vi "_Get Experiment List.vi"(4 "error in (no error)":errorcluster, 7 "node in":refnum<k20>) -> (0 "error out":errorcluster, 1 "ExptParamAndMR":T2(array[cluster]), 2 "Expt":string[][](array[string]), 3 "node out":refnum<k20>)   [LabVIEW 2015]
uses:
  Type/_Mass Range Parameters.ctl
  Server/AutoCal/Controls/xml Parameter Type.ctl
  <vilib>/xml/Close Reference(Node).vi
  <vilib>/xml/NI_XML.lvlib
panel:
  # "Num             Type            Polarity        StartTime      StopTime        Cycles       PauseTime    DelayTime          MR#         DwellTime   Comment"
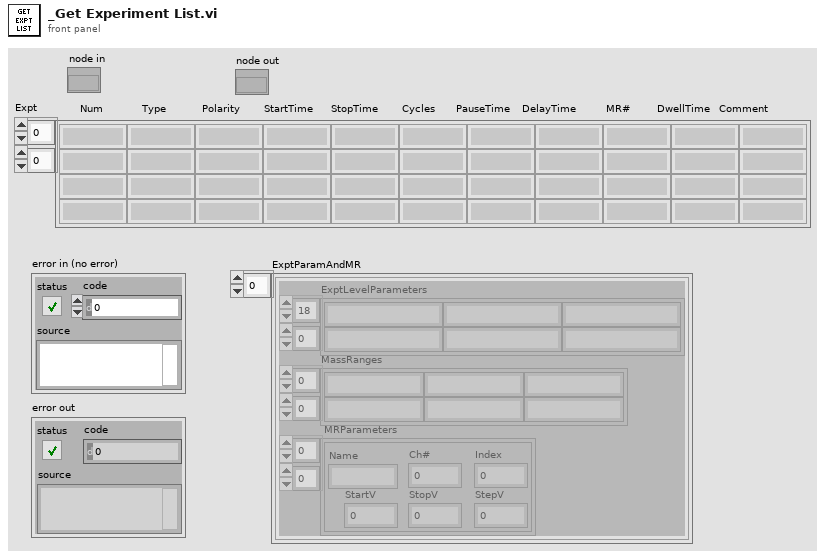
[diagram p1: front panel]
types:
  T1 = typedef "_Mass Range Parameters.ctl" = cluster{"Name":string, "Ch#":u8, "StartV":dbl, "StopV":dbl, "StepV":dbl, "Index":u8}
  T2 = cluster{"ExptLevelParameters":string[][], "MassRanges":string[][], " MRParameters":T1[][]}[]
  T3 = typedef "xml Parameter Type.ctl" = enum16{"Method Parameters", "Experiment Parameters"}
  T4 = cluster{"Parameters List":string[][], "Mass Ranges":string[][], " MRParameters":T1[][]}
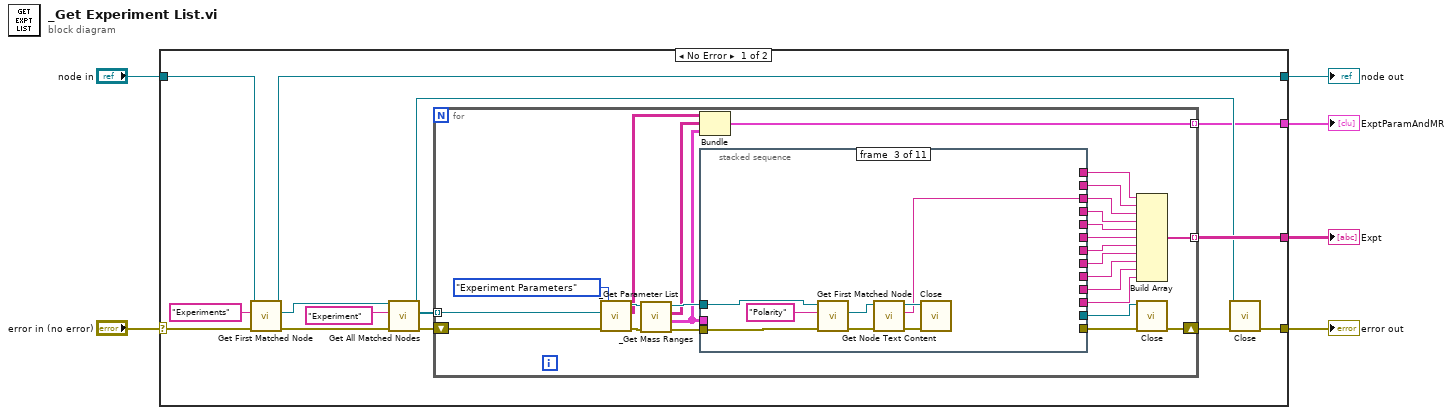
[diagram p0: block diagram]
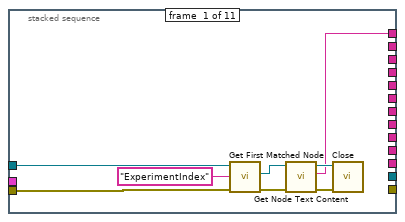
[diagram p2: hidden frame]
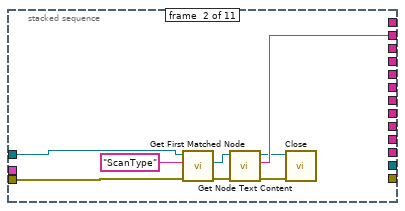
[diagram p3: hidden frame]
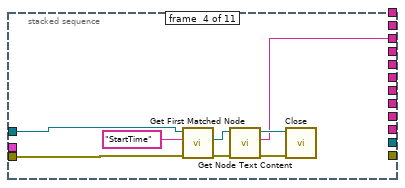
[diagram p4: hidden frame]
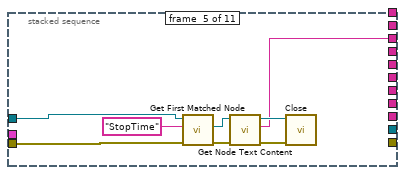
[diagram p5: hidden frame]
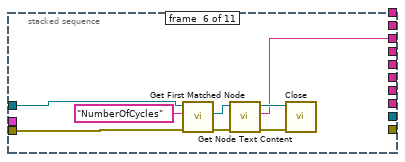
[diagram p6: hidden frame]
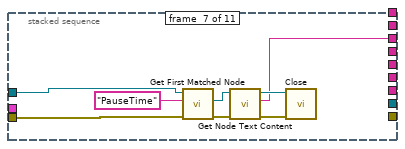
[diagram p7: hidden frame]
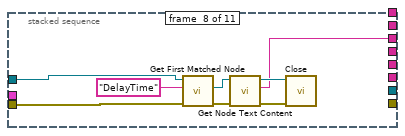
[diagram p8: hidden frame]
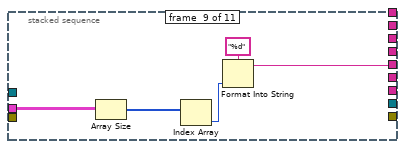
[diagram p9: hidden frame]
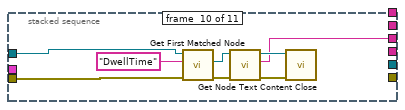
[diagram p10: hidden frame]
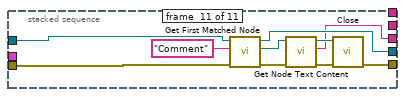
[diagram p11: hidden frame]
diagram:
  n1 = case shown="No Error" "error in (no error)" {
    selector: "error in (no error)" -> [w18 w135]
    tunnel: [w19 _] -> w6
    tunnel: [w9 w135] -> w5
    tunnel: "node in" -> [w16 w134]
    tunnel: [w15 w134] -> w2
    tunnel: [w7 _] -> w1
    frame No Error {
      n2 = call <vilib>:"Get First Matched Node.vi"("error in (no error)"=w18, "XPath expression"="Experiments", "node in"=w16) -> ("error out"=w17:errorcluster, "node result"=w13:refnum<k20>, "node out"=w15:refnum<k20>)  [unwired: 6 in]
      n3 = call <vilib>:"Get All Matched Nodes.vi"("error in (no error)"=w17, "XPath expression"="Experiment", "node in"=w13) -> ("error out"=w11:errorcluster, "node result array"=w12:refnum<k20>[], "node out"=w8:refnum<k20>)  [unwired: 6 in]
      n4 = for {
        shift-right: [w46] -> w10
        shift-left: w11 -> [w30]
        tunnel: w12 -> [w31] mode=indexing
        tunnel: [w36] -> w19 mode=indexing
        tunnel: [w23] -> w7 mode=indexing
        n5 = call "_Get Parameter List.vi"("error in (no error)"=w30, "Parameter Type"=xml_Parameter_Type."Experiment Parameters", "node in"=w31) -> ("error out"=w27:errorcluster, "Parameters List"=w25:string[][], "node out"=w29:refnum<k20>)  [unwired: 2 in]
        n6 = call "_Get Mass Ranges.vi"("error in (no error)"=w27, "node in"=w29) -> ("error out"=w26:errorcluster, "MRParameters"=w21:T1[][], "Mass Ranges"=w24:string[][], "node out"=w28:refnum<k20>)  [unwired: 2 in]
        n7 = Bundle("Parameters List"=w25, "Mass Ranges"=w24, "MRParameters"=w21) -> (w23:T4)  [unwired: 1 in]
        n8 = stacked-sequence {
          tunnel: w28 -> [w54 w62 w70 w78 w86 w94 w102 w110 _ w123 w133]
          tunnel: w26 -> [w53 w61 w69 w77 w85 w93 w101 w109 _ w122 w132]
          tunnel: [w47 _ _ _ _ _ _ _ _ _ _] -> w45
          tunnel: [_ w58 _ _ _ _ _ _ _ _ _] -> w44
          tunnel: [_ _ w63 _ _ _ _ _ _ _ _] -> w43
          tunnel: [_ _ _ w71 _ _ _ _ _ _ _] -> w42
          tunnel: [_ _ _ _ w79 _ _ _ _ _ _] -> w41
          tunnel: [_ _ _ _ _ w87 _ _ _ _ _] -> w40
          tunnel: [_ _ _ _ _ _ w95 _ _ _ _] -> w39
          tunnel: [_ _ _ _ _ _ _ w103 _ _ _] -> w38
          tunnel: [_ _ _ _ _ _ _ _ w111 _ _] -> w37
          tunnel: [_ _ _ _ _ _ _ _ _ _ w130] -> w35
          tunnel: [_ _ _ _ _ _ _ _ _ _ w129] -> w34
          tunnel: [_ _ _ _ _ _ _ _ _ _ w124] -> w33
          tunnel: [_ _ _ _ _ _ _ _ _ w116 _] -> w32
          tunnel: w21 -> [_ _ _ _ _ _ _ _ w115 _ _]
          frame #0 {
            n9 = call <vilib>:"Get First Matched Node.vi"("error in (no error)"=w53, "XPath expression"="ExperimentIndex", "node in"=w54) -> ("error out"=w50:errorcluster, "node result"=w51:refnum<k20>)  [unwired: 6 in, 1 out]
            n10 = call <vilib>:"Get Node Text Content.vi"("error in (no error)"=w50, "node in"=w51) -> ("error out"=w48:errorcluster, "node text"=w47:string, "node out"=w49:refnum<k20>)  [unwired: 7 in]
            n11 = call-poly <vilib>:"Close.vi"("error in (no error)"=w48, "node"=w49) -> ()  [unwired: 7 in, 1 out]
          }
          frame #1 {
            n12 = call <vilib>:"Get First Matched Node.vi"("error in (no error)"=w61, "XPath expression"="ScanType", "node in"=w62) -> ("error out"=w55:errorcluster, "node result"=w59:refnum<k20>)  [unwired: 6 in, 1 out]
            n13 = call <vilib>:"Get Node Text Content.vi"("error in (no error)"=w55, "node in"=w59) -> ("error out"=w56:errorcluster, "node text"=w58:string, "node out"=w57:refnum<k20>)  [unwired: 7 in]
            n14 = call-poly <vilib>:"Close.vi"("error in (no error)"=w56, "node"=w57) -> ()  [unwired: 7 in, 1 out]
          }
          frame #2 {
            n15 = call <vilib>:"Get First Matched Node.vi"("error in (no error)"=w69, "XPath expression"="Polarity", "node in"=w70) -> ("error out"=w66:errorcluster, "node result"=w67:refnum<k20>)  [unwired: 6 in, 1 out]
            n16 = call <vilib>:"Get Node Text Content.vi"("error in (no error)"=w66, "node in"=w67) -> ("error out"=w65:errorcluster, "node text"=w63:string, "node out"=w64:refnum<k20>)  [unwired: 7 in]
            n17 = call-poly <vilib>:"Close.vi"("error in (no error)"=w65, "node"=w64) -> ()  [unwired: 7 in, 1 out]
          }
          frame #3 {
            n18 = call <vilib>:"Get First Matched Node.vi"("error in (no error)"=w77, "XPath expression"="StartTime", "node in"=w78) -> ("error out"=w74:errorcluster, "node result"=w75:refnum<k20>)  [unwired: 6 in, 1 out]
            n19 = call <vilib>:"Get Node Text Content.vi"("error in (no error)"=w74, "node in"=w75) -> ("error out"=w72:errorcluster, "node text"=w71:string, "node out"=w73:refnum<k20>)  [unwired: 7 in]
            n20 = call-poly <vilib>:"Close.vi"("error in (no error)"=w72, "node"=w73) -> ()  [unwired: 7 in, 1 out]
          }
          frame #4 {
            n21 = call <vilib>:"Get First Matched Node.vi"("error in (no error)"=w85, "XPath expression"="StopTime", "node in"=w86) -> ("error out"=w81:errorcluster, "node result"=w83:refnum<k20>)  [unwired: 6 in, 1 out]
            n22 = call <vilib>:"Get Node Text Content.vi"("error in (no error)"=w81, "node in"=w83) -> ("error out"=w80:errorcluster, "node text"=w79:string, "node out"=w82:refnum<k20>)  [unwired: 7 in]
            n23 = call-poly <vilib>:"Close.vi"("error in (no error)"=w80, "node"=w82) -> ()  [unwired: 7 in, 1 out]
          }
          frame #5 {
            n24 = call <vilib>:"Get First Matched Node.vi"("error in (no error)"=w93, "XPath expression"="NumberOfCycles", "node in"=w94) -> ("error out"=w89:errorcluster, "node result"=w91:refnum<k20>)  [unwired: 6 in, 1 out]
            n25 = call <vilib>:"Get Node Text Content.vi"("error in (no error)"=w89, "node in"=w91) -> ("error out"=w88:errorcluster, "node text"=w87:string, "node out"=w90:refnum<k20>)  [unwired: 7 in]
            n26 = call-poly <vilib>:"Close.vi"("error in (no error)"=w88, "node"=w90) -> ()  [unwired: 7 in, 1 out]
          }
          frame #6 {
            n27 = call <vilib>:"Get First Matched Node.vi"("error in (no error)"=w101, "XPath expression"="PauseTime", "node in"=w102) -> ("error out"=w98:errorcluster, "node result"=w99:refnum<k20>)  [unwired: 6 in, 1 out]
            n28 = call <vilib>:"Get Node Text Content.vi"("error in (no error)"=w98, "node in"=w99) -> ("error out"=w97:errorcluster, "node text"=w95:string, "node out"=w96:refnum<k20>)  [unwired: 7 in]
            n29 = call-poly <vilib>:"Close.vi"("error in (no error)"=w97, "node"=w96) -> ()  [unwired: 7 in, 1 out]
          }
          frame #7 {
            n30 = call <vilib>:"Get First Matched Node.vi"("error in (no error)"=w109, "XPath expression"="DelayTime", "node in"=w110) -> ("error out"=w106:errorcluster, "node result"=w107:refnum<k20>)  [unwired: 6 in, 1 out]
            n31 = call <vilib>:"Get Node Text Content.vi"("error in (no error)"=w106, "node in"=w107) -> ("error out"=w104:errorcluster, "node text"=w103:string, "node out"=w105:refnum<k20>)  [unwired: 7 in]
            n32 = call-poly <vilib>:"Close.vi"("error in (no error)"=w104, "node"=w105) -> ()  [unwired: 7 in, 1 out]
          }
          frame #8 {
            n33 = Array Size(array=w115) -> (size(s)=w114:i32[])
            n34 = Index Array(array=w114) -> (element=w113:i32)  [unwired: 1 in]
            n35 = Format Into String(format string="%d", w113) -> (resulting string=w111:string)  [unwired: 2 in, 1 out]
          }
          frame #9 {
            n36 = call <vilib>:"Get First Matched Node.vi"("error in (no error)"=w122, "XPath expression"="DwellTime", "node in"=w123) -> ("error out"=w117:errorcluster, "node result"=w120:refnum<k20>)  [unwired: 6 in, 1 out]
            n37 = call <vilib>:"Get Node Text Content.vi"("error in (no error)"=w117, "node in"=w120) -> ("error out"=w118:errorcluster, "node text"=w116:string, "node out"=w119:refnum<k20>)  [unwired: 7 in]
            n38 = call-poly <vilib>:"Close.vi"("error in (no error)"=w118, "node"=w119) -> ()  [unwired: 7 in, 1 out]
          }
          frame #10 {
            n39 = call <vilib>:"Get First Matched Node.vi"("error in (no error)"=w132, "XPath expression"="Comment", "node in"=w133) -> ("error out"=w127:errorcluster, "node result"=w128:refnum<k20>, "node out"=w130:refnum<k20>)  [unwired: 6 in]
            n40 = call <vilib>:"Get Node Text Content.vi"("error in (no error)"=w127, "node in"=w128) -> ("error out"=w125:errorcluster, "node text"=w124:string, "node out"=w126:refnum<k20>)  [unwired: 7 in]
            n41 = call-poly <vilib>:"Close.vi"("error in (no error)"=w125, "node"=w126) -> ("error out"=w129:errorcluster)  [unwired: 7 in]
          }
        }
        n42 = Build Array(w45, w44, w43, w42, w41, w40, w39, w38, w37, w32, w33) -> (w36:string[])
        n43 = call-poly <vilib>:"Close.vi"("error in (no error)"=w34, "node"=w35) -> ("error out"=w46:errorcluster)  [unwired: 7 in]
      }
      n44 = call-poly <vilib>:"Close.vi"("error in (no error)"=w10, "node"=w8) -> ("error out"=w9:errorcluster)  [unwired: 7 in]
    }
    frame Error {
    }
  }
  "Expt" <- w6
  "error out" <- w5
  "node out" <- w2
  "ExptParamAndMR" <- w1
